vi "读取反控数据解析(子VI).vi"(6 "数据":string, 7 "命令编码CN":string) -> (2 "设置超时时间/min":i32=1, 3 "反控命令错误？":bool)   [LabVIEW 2016, in "数据传输系统-06.lvlib"]
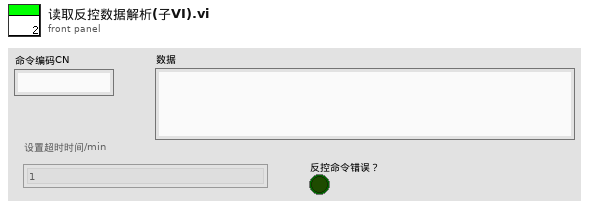
[diagram p1: front panel]
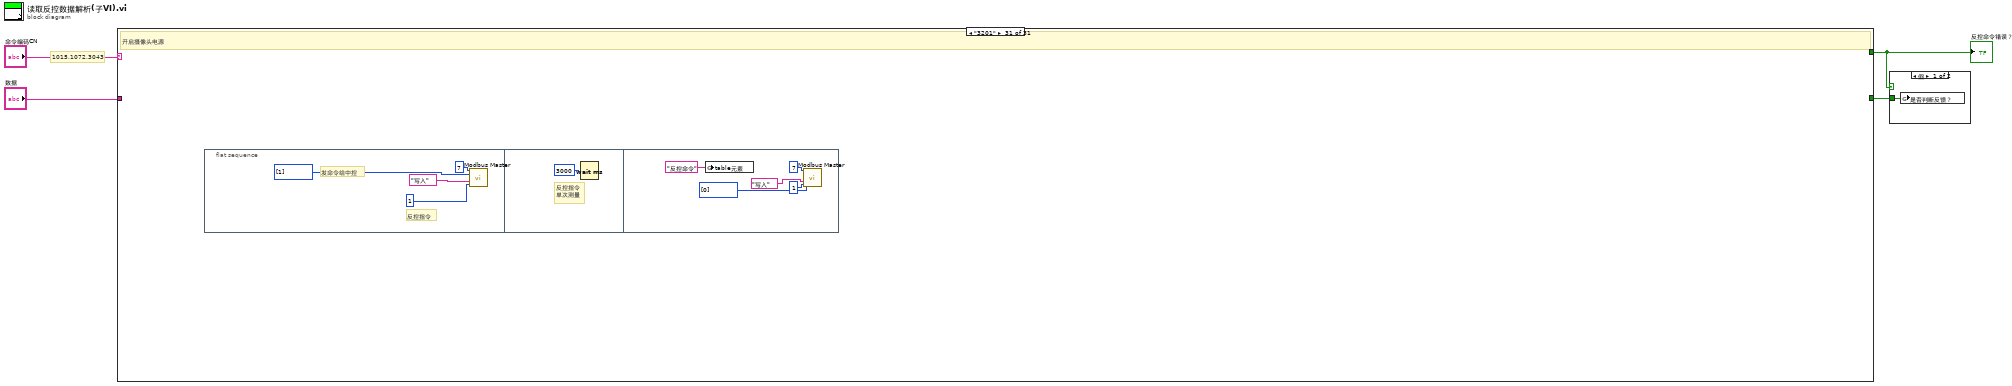
[diagram p0: block diagram]
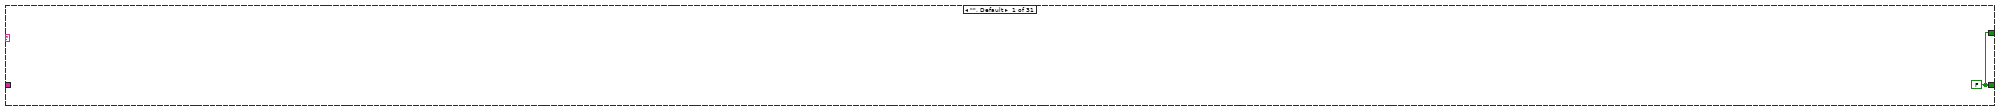
[diagram p2: hidden frame]
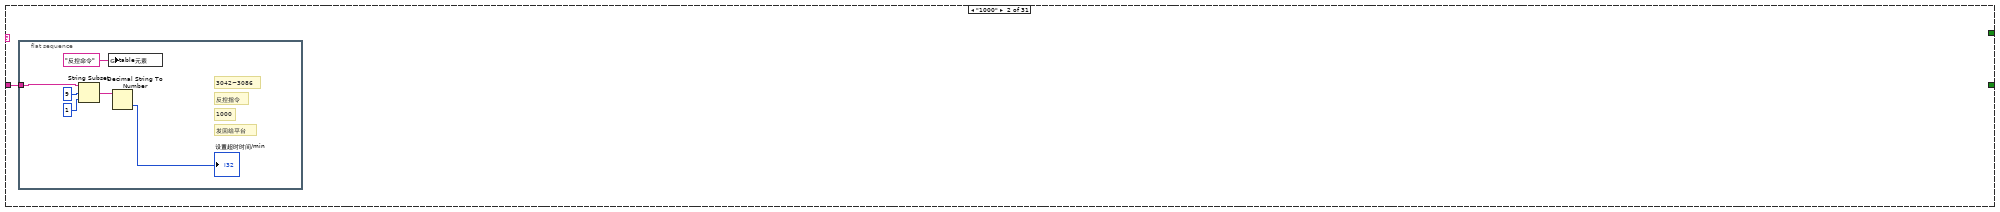
[diagram p3: hidden frame]
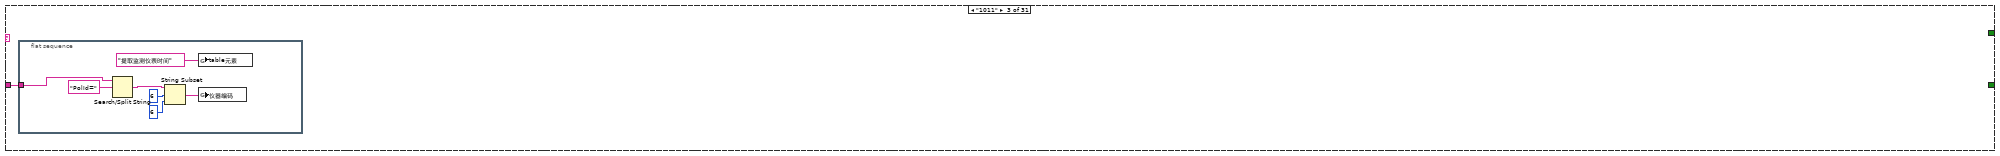
[diagram p4: hidden frame]
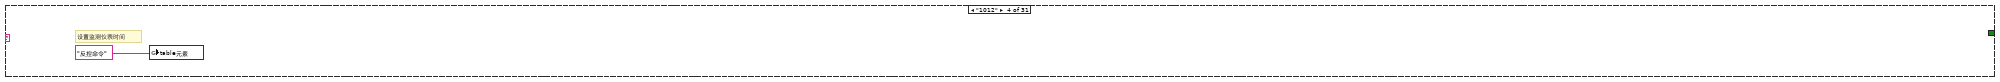
[diagram p5: hidden frame]
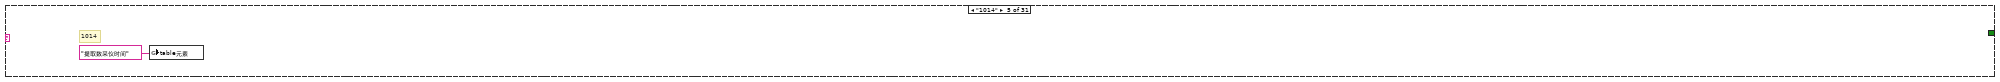
[diagram p6: hidden frame]
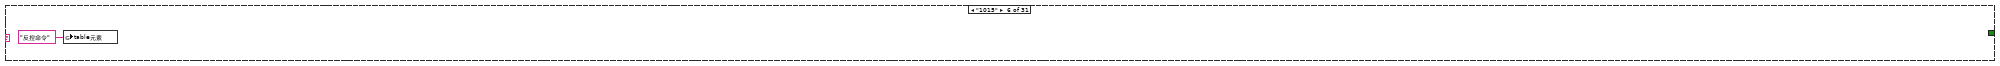
[diagram p7: hidden frame]
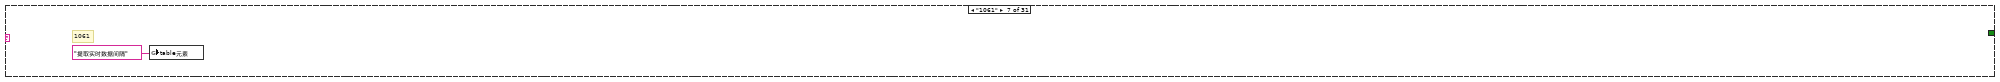
[diagram p8: hidden frame]
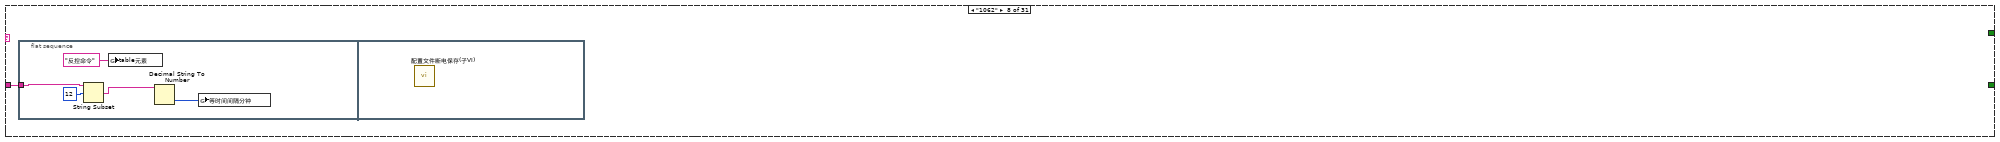
[diagram p9: hidden frame]
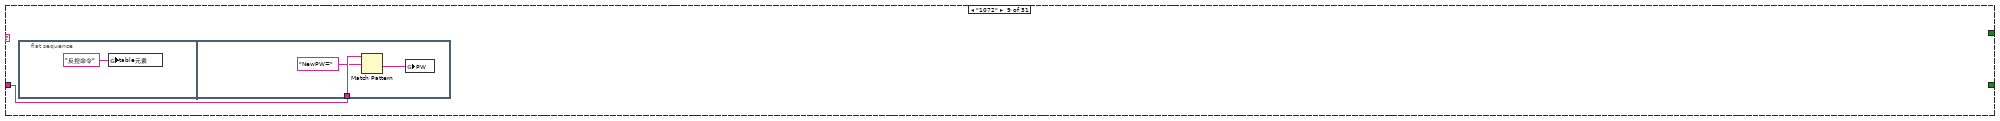
[diagram p10: hidden frame]
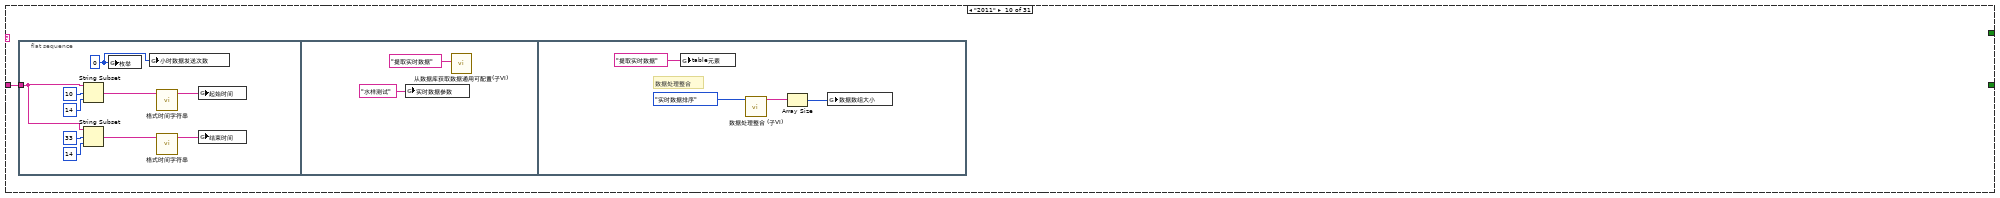
[diagram p11: hidden frame]
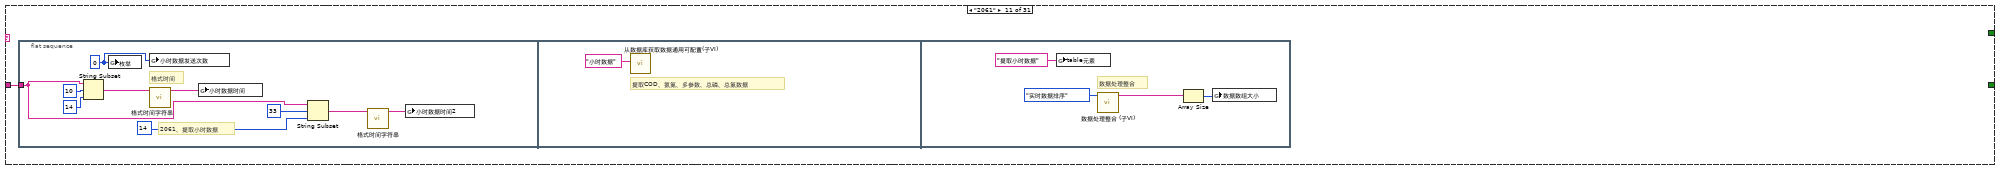
[diagram p12: hidden frame]
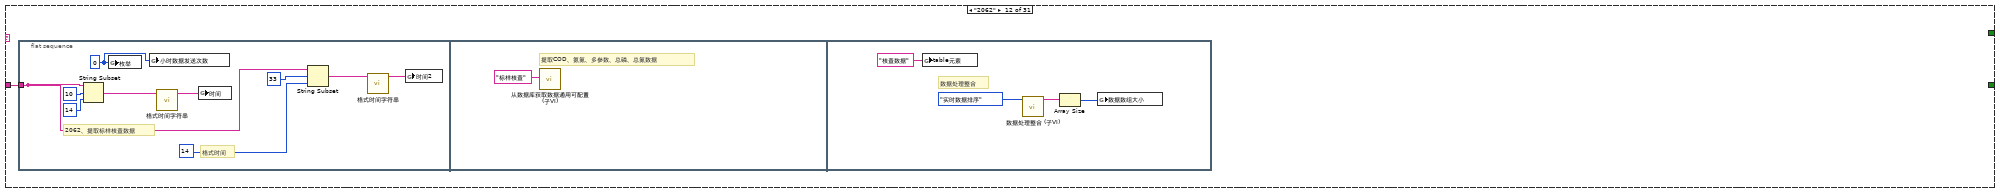
[diagram p13: hidden frame]
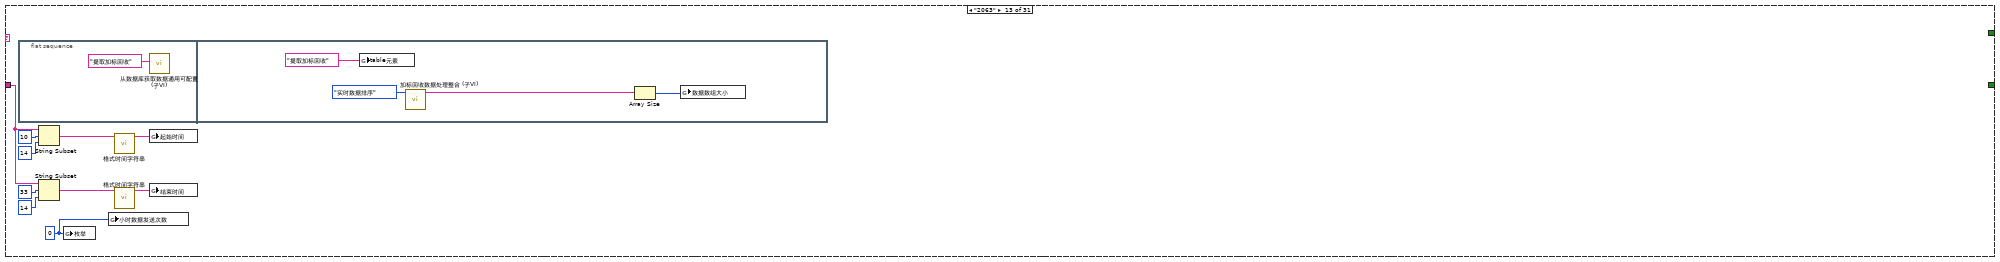
[diagram p14: hidden frame]
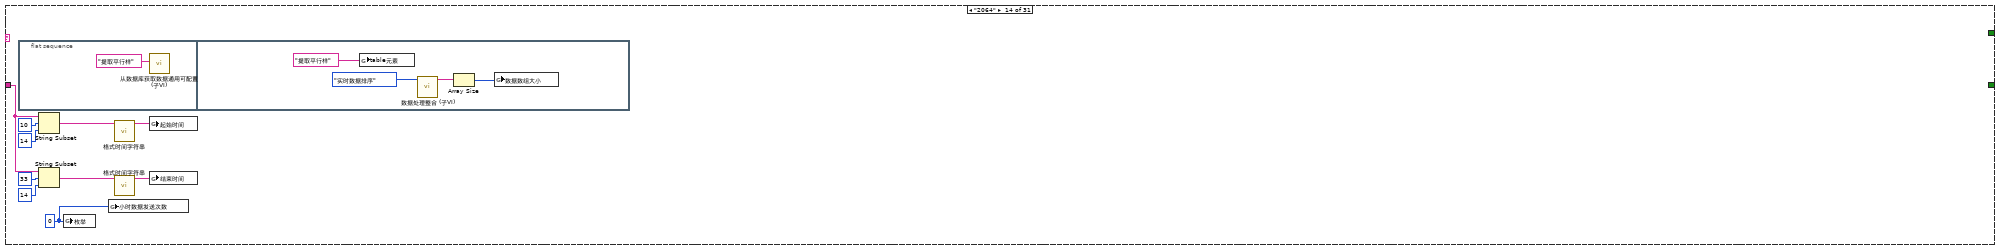
[diagram p15: hidden frame]
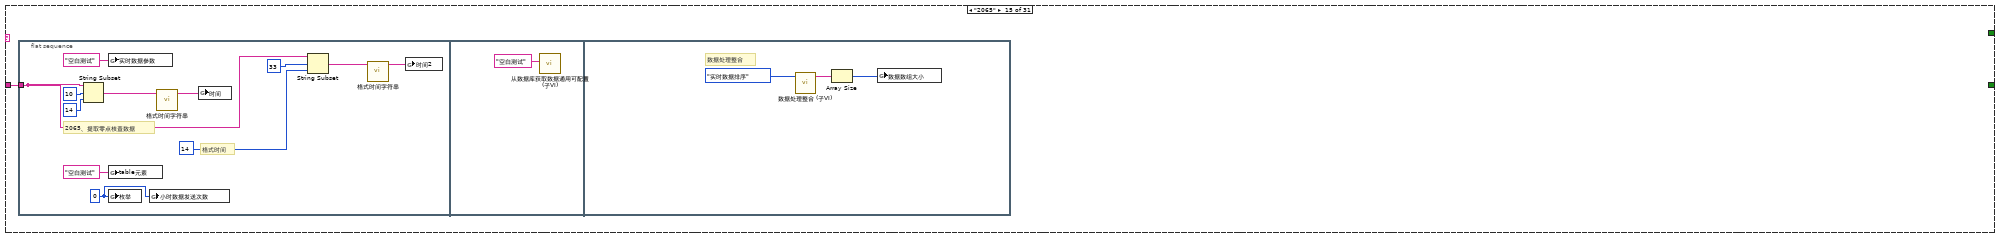
[diagram p16: hidden frame]
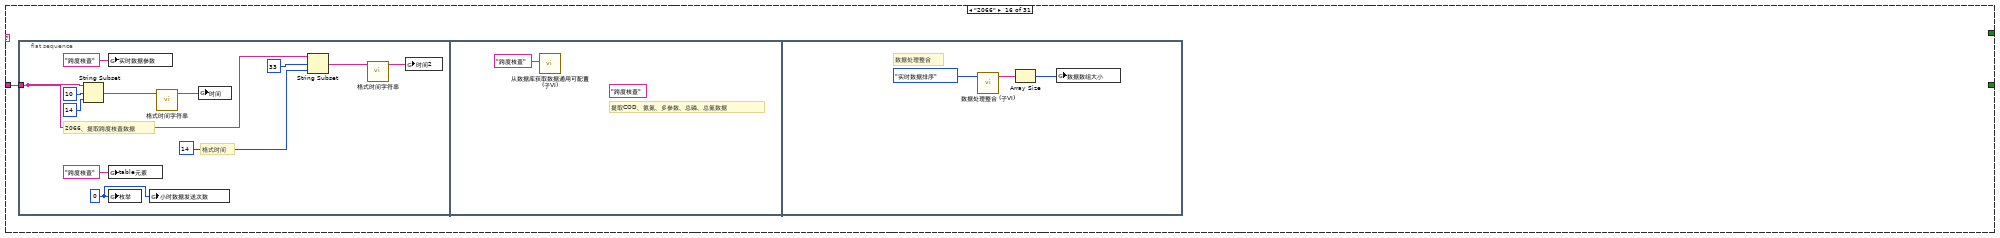
[diagram p17: hidden frame]
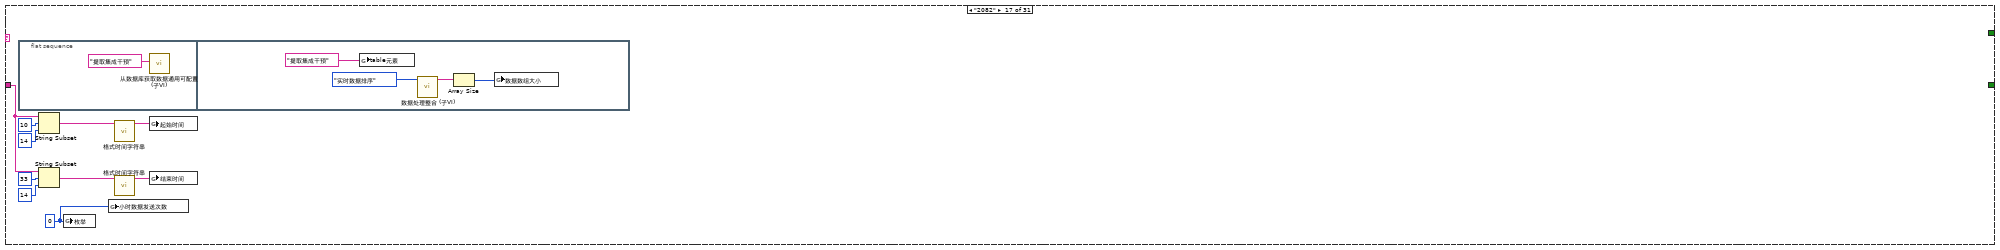
[diagram p18: hidden frame]
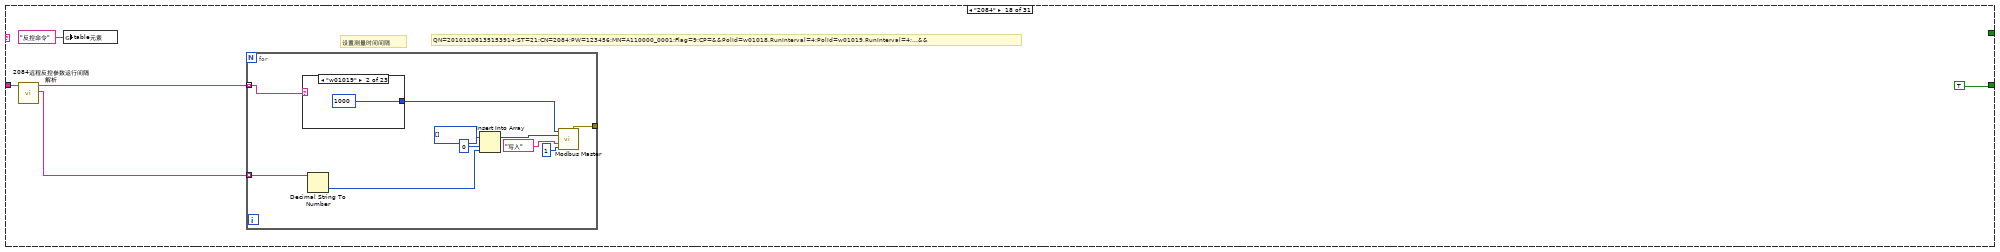
[diagram p19: hidden frame]
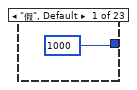
[diagram p20: hidden frame]
diagram:
  # "1015,1072,3043"
  n1 = case shown="\"3201\"" "命令编码CN" {
    selector: "命令编码CN" -> [_ _ _ _ _ _ _ _ _ _ _ _ _ _ _ _ _ _ _ _ _ _ _ _ _ _ _ _ w499 _ _]
    tunnel: "数据" -> [_ w6 w13 _ _ _ _ w25 w31 w36 w53 w69 w86 w100 w115 w132 w149 w165 _ w210 w367 _ _ w459 _ _ _ w498 w500 _ _]
    tunnel: [w5 _ _ _ _ _ _ _ _ _ _ _ _ _ _ _ _ _ _ _ _ _ _ _ _ _ _ _ _ _ _] -> w2
    tunnel: [w5 _ _ _ _ _ _ _ _ _ _ _ _ _ _ _ _ TRUE _ _ TRUE _ _ TRUE ("是否判断反馈？") _ _ _ _ TRUE _ _] -> w1
    frame "", Default {
      w5 = FALSE
    }
    frame "1000" {
      n2 = flat-sequence {
        tunnel: w6 -> [w8]
        frame #0 {
          # "发回给平台"
          # "3042~3086"
          # "反控指令"
          # "1000"
          n3 = String Subset(string=w8, offset (0)=9 ("偏移量(0)"), length (rest)=1 ("长度（剩余）")) -> (substring=w10:string)
          n4 = global write "全局1.vi" "table元素"("反控命令" ("新元素/子数组")) -> ()
          n5 = Decimal String To Number(string=w10) -> (number=→"设置超时时间/min":i32)  [unwired: 2 in, 1 out]
        }
      }
    }
    frame "1011" {
      n6 = flat-sequence {
        tunnel: w13 -> [w14]
        frame #0 {
          n7 = Search/Split String(string=w14, search string/char (-)="PolId=" ("搜索字符串/字符(-)")) -> (match + rest of string=w19:string)  [unwired: 1 in, 2 out]
          n8 = String Subset(string=w19, offset (0)=6 ("偏移量(0)"), length (rest)=6 ("长度（剩余）")) -> (substring=w16:string)
          n9 = global write "全局1.vi" "table元素"("提取监测仪表时间") -> ()
          n10 = global write "全局 提取仪器参数.vi" "仪器编码"(w16) -> ()
        }
      }
    }
    frame "1012" {
      # "设置监测仪表时间"
      n11 = global write "全局1.vi" "table元素"("反控命令" ("新元素/子数组")) -> ()
    }
    frame "1014" {
      # "1014"
      n12 = global write "全局1.vi" "table元素"("提取数采仪时间") -> ()
    }
    frame "1015" {
      n13 = global write "全局1.vi" "table元素"("反控命令" ("新元素/子数组")) -> ()
    }
    frame "1061" {
      # "1061"
      n14 = global write "全局1.vi" "table元素"("提取实时数据间隔") -> ()
    }
    frame "1062" {
      n15 = flat-sequence {
        tunnel: w25 -> [w28]
        frame #0 {
          n16 = String Subset(string=w28, offset (0)=12 ("偏移量(0)")) -> (substring=w29:string)  [unwired: 1 in]
          n17 = global write "全局1.vi" "table元素"("反控命令" ("新元素/子数组")) -> ()
          n18 = Decimal String To Number(string=w29) -> (number=w26:i32)  [unwired: 2 in, 1 out]
          n19 = global write "断电保存全局.vi" "等时间间隔分钟"(w26) -> ()
        }
        frame #1 {
          n20 = call "配置文件断电保存(子VI).vi"() -> ()  [unwired: 12 in]
        }
      }
    }
    frame "1072" {
      n21 = flat-sequence {
        tunnel: w31 -> [w35]
        frame #0 {
          n22 = global write "全局1.vi" "table元素"("反控命令" ("新元素/子数组")) -> ()
        }
        frame #1 {
          n23 = Match Pattern(string=w35, regular expression="NewPW=" ("正则表达式")) -> (after substring=w33:string)  [unwired: 1 in, 3 out]
          n24 = global write "断电保存全局.vi" "PW"(w33) -> ()
        }
      }
    }
    frame "2011" {
      n25 = flat-sequence {
        tunnel: w36 -> [w37]
        frame #0 {
          w42 = 0 ("数值")
          n26 = String Subset(string=w37, offset (0)=10 ("偏移量(0)"), length (rest)=14 ("长度（剩余）")) -> (substring=w45:string)
          n27 = String Subset(string=w37, offset (0)=33 ("偏移量(0)"), length (rest)=14 ("长度（剩余）")) -> (substring=w43:string)
          n28 = global write "全局1.vi" "枚举"(w42) -> ()
          n29 = global write "全局 小时数据发送次数.vi" "小时数据发送次数"(w42) -> ()
          n30 = call "格式时间字符串.vi"("字符串"=w45) -> ("连接的字符串"=w46:string)  [unwired: 10 in]
          n31 = call "格式时间字符串.vi"("字符串"=w43) -> ("连接的字符串"=w44:string)  [unwired: 10 in]
          n32 = global write "起始时间.vi" "起始时间"(w46) -> ()
          n33 = global write "起始时间.vi" "结束时间"(w44) -> ()
        }
        frame #1 {
          n34 = global write "全局 实时数据参数.vi" "实时数据参数"("水样测试") -> ()
          n35 = call "从数据库获取数据通用可配置(子VI).vi"("table输入"="提取实时数据" ("新元素/子数组")) -> ()  [unwired: 9 in, 2 out]
        }
        frame #2 {
          # "数据处理整合"
          n36 = global write "全局1.vi" "table元素"("提取实时数据" ("新元素/子数组")) -> ()
          n37 = call "数据处理整合 (子VI).vi"("枚举"=enum16{"实时数据排序", "小时数据排序"}."实时数据排序") -> ("已排序的数组"=w51:string[])  [unwired: 10 in]
          n38 = Array Size(array=w51) -> (size(s)=w52:i32)
          n39 = global write "全局 数据数组大小.vi" "数据数组大小"(w52) -> ()
        }
      }
    }
    frame "2061" {
      n40 = flat-sequence {
        tunnel: w53 -> [w54]
        frame #0 {
          w55 = 0 ("数值")
          # "格式时间"
          # "2061、提取小时数据"
          n41 = String Subset(string=w54, offset (0)=10 ("偏移量(0)"), length (rest)=14 ("长度（剩余）")) -> (substring=w58:string)
          n42 = global write "全局1.vi" "枚举"(w55) -> ()
          n43 = global write "全局 小时数据发送次数.vi" "小时数据发送次数"(w55) -> ()
          n44 = call "格式时间字符串.vi"("字符串"=w58) -> ("连接的字符串"=w59:string)  [unwired: 10 in]
          n45 = global write "全局 水样时间.vi" "小时数据时间"(w59) -> ()
          n46 = String Subset(string=w54, offset (0)=33 ("偏移量(0)"), length (rest)=14 ("长度（剩余）")) -> (substring=w57:string)
          n47 = call "格式时间字符串.vi"("字符串"=w57) -> ("连接的字符串"=w56:string)  [unwired: 10 in]
          n48 = global write "全局 时间2.vi" "小时数据时间2"(w56) -> ()
        }
        frame #1 {
          # "提取COD、氨氮、多参数、总磷、总氮数据"
          n49 = call "从数据库获取数据通用可配置(子VI).vi"("table输入"="小时数据" ("名称（未命名）")) -> ()  [unwired: 9 in, 2 out]
        }
        frame #2 {
          # "数据处理整合"
          n50 = global write "全局1.vi" "table元素"("提取小时数据" ("新元素/子数组")) -> ()
          n51 = call "数据处理整合 (子VI).vi"("枚举"=enum16{"实时数据排序", "小时数据排序"}."实时数据排序") -> ("已排序的数组"=w68:string[])  [unwired: 10 in]
          n52 = Array Size(array=w68) -> (size(s)=w67:i32)
          n53 = global write "全局 数据数组大小.vi" "数据数组大小"(w67) -> ()
        }
      }
    }
    frame "2062" {
      n54 = flat-sequence {
        tunnel: w69 -> [w70]
        frame #0 {
          w71 = 0 ("数值")
          # "格式时间"
          # "2062、提取标样核查数据"
          n55 = String Subset(string=w70, offset (0)=10 ("偏移量(0)"), length (rest)=14 ("长度（剩余）")) -> (substring=w74:string)
          n56 = global write "全局1.vi" "枚举"(w71) -> ()
          n57 = global write "全局 小时数据发送次数.vi" "小时数据发送次数"(w71) -> ()
          n58 = call "格式时间字符串.vi"("字符串"=w74) -> ("连接的字符串"=w75:string)  [unwired: 10 in]
          n59 = global write "全局 水样时间.vi" "时间"(w75) -> ()
          n60 = String Subset(string=w70, offset (0)=33 ("偏移量(0)"), length (rest)=14 ("长度（剩余）")) -> (substring=w73:string)
          n61 = call "格式时间字符串.vi"("字符串"=w73) -> ("连接的字符串"=w72:string)  [unwired: 10 in]
          n62 = global write "全局 时间2.vi" "时间2"(w72) -> ()
        }
        frame #1 {
          # "提取COD、氨氮、多参数、总磷、总氮数据"
          n63 = call "从数据库获取数据通用可配置(子VI).vi"("table输入"="标样核查" ("新元素/子数组")) -> ()  [unwired: 9 in, 2 out]
        }
        frame #2 {
          # "数据处理整合"
          n64 = global write "全局1.vi" "table元素"("核查数据" ("新元素/子数组")) -> ()
          n65 = call "数据处理整合 (子VI).vi"("枚举"=enum16{"实时数据排序", "小时数据排序"}."实时数据排序") -> ("已排序的数组"=w83:string[])  [unwired: 10 in]
          n66 = Array Size(array=w83) -> (size(s)=w84:i32)
          n67 = global write "全局 数据数组大小.vi" "数据数组大小"(w84) -> ()
        }
      }
    }
    frame "2063" {
      w85 = 0 ("数值")
      n68 = flat-sequence {
        frame #0 {
          n69 = call "从数据库获取数据通用可配置(子VI).vi"("table输入"="提取加标回收" ("新元素/子数组")) -> ()  [unwired: 9 in, 2 out]
        }
        frame #1 {
          n70 = global write "全局1.vi" "table元素"("提取加标回收" ("新元素/子数组")) -> ()
          n71 = call "加标回收数据处理整合 (子VI).vi"("枚举"=enum16{"实时数据排序", "小时数据排序"}."实时数据排序") -> ("已排序的数组"=w97:string[])  [unwired: 10 in]
          n72 = Array Size(array=w97) -> (size(s)=w99:i32)
          n73 = global write "全局 数据数组大小.vi" "数据数组大小"(w99) -> ()
        }
      }
      n74 = String Subset(string=w86, offset (0)=10 ("偏移量(0)"), length (rest)=14 ("长度（剩余）")) -> (substring=w88:string)
      n75 = String Subset(string=w86, offset (0)=33 ("偏移量(0)"), length (rest)=14 ("长度（剩余）")) -> (substring=w90:string)
      n76 = global write "全局1.vi" "枚举"(w85) -> ()
      n77 = global write "全局 小时数据发送次数.vi" "小时数据发送次数"(w85) -> ()
      n78 = call "格式时间字符串.vi"("字符串"=w88) -> ("连接的字符串"=w87:string)  [unwired: 10 in]
      n79 = call "格式时间字符串.vi"("字符串"=w90) -> ("连接的字符串"=w89:string)  [unwired: 10 in]
      n80 = global write "起始时间.vi" "起始时间"(w87) -> ()
      n81 = global write "起始时间.vi" "结束时间"(w89) -> ()
    }
    frame "2064" {
      w105 = 0 ("数值")
      n82 = flat-sequence {
        frame #0 {
          n83 = call "从数据库获取数据通用可配置(子VI).vi"("table输入"="提取平行样" ("新元素/子数组")) -> ()  [unwired: 9 in, 2 out]
        }
        frame #1 {
          n84 = global write "全局1.vi" "table元素"("提取平行样" ("新元素/子数组")) -> ()
          n85 = call "数据处理整合 (子VI).vi"("枚举"=enum16{"实时数据排序", "小时数据排序"}."实时数据排序") -> ("已排序的数组"=w114:string[])  [unwired: 10 in]
          n86 = Array Size(array=w114) -> (size(s)=w113:i32)
          n87 = global write "全局 数据数组大小.vi" "数据数组大小"(w113) -> ()
        }
      }
      n88 = String Subset(string=w100, offset (0)=10 ("偏移量(0)"), length (rest)=14 ("长度（剩余）")) -> (substring=w108:string)
      n89 = String Subset(string=w100, offset (0)=33 ("偏移量(0)"), length (rest)=14 ("长度（剩余）")) -> (substring=w106:string)
      n90 = global write "全局1.vi" "枚举"(w105) -> ()
      n91 = global write "全局 小时数据发送次数.vi" "小时数据发送次数"(w105) -> ()
      n92 = call "格式时间字符串.vi"("字符串"=w108) -> ("连接的字符串"=w109:string)  [unwired: 10 in]
      n93 = call "格式时间字符串.vi"("字符串"=w106) -> ("连接的字符串"=w107:string)  [unwired: 10 in]
      n94 = global write "起始时间.vi" "起始时间"(w109) -> ()
      n95 = global write "起始时间.vi" "结束时间"(w107) -> ()
    }
    frame "2065" {
      n96 = flat-sequence {
        tunnel: w115 -> [w117]
        frame #0 {
          w118 = 0 ("数值")
          # "格式时间"
          # "2065、提取零点核查数据"
          n97 = String Subset(string=w117, offset (0)=10 ("偏移量(0)"), length (rest)=14 ("长度（剩余）")) -> (substring=w122:string)
          n98 = global write "全局 实时数据参数.vi" "实时数据参数"("空白测试" ("新元素/子数组")) -> ()
          n99 = global write "全局1.vi" "table元素"("空白测试" ("新元素/子数组")) -> ()
          n100 = global write "全局1.vi" "枚举"(w118) -> ()
          n101 = global write "全局 小时数据发送次数.vi" "小时数据发送次数"(w118) -> ()
          n102 = call "格式时间字符串.vi"("字符串"=w122) -> ("连接的字符串"=w123:string)  [unwired: 10 in]
          n103 = global write "全局 水样时间.vi" "时间"(w123) -> ()
          n104 = String Subset(string=w117, offset (0)=33 ("偏移量(0)"), length (rest)=14 ("长度（剩余）")) -> (substring=w121:string)
          n105 = call "格式时间字符串.vi"("字符串"=w121) -> ("连接的字符串"=w120:string)  [unwired: 10 in]
          n106 = global write "全局 时间2.vi" "时间2"(w120) -> ()
        }
        frame #1 {
          n107 = call "从数据库获取数据通用可配置(子VI).vi"("table输入"="空白测试" ("新元素/子数组")) -> ()  [unwired: 9 in, 2 out]
        }
        frame #2 {
          # "数据处理整合"
          n108 = call "数据处理整合 (子VI).vi"("枚举"=enum16{"实时数据排序", "小时数据排序"}."实时数据排序") -> ("已排序的数组"=w130:string[])  [unwired: 10 in]
          n109 = Array Size(array=w130) -> (size(s)=w131:i32)
          n110 = global write "全局 数据数组大小.vi" "数据数组大小"(w131) -> ()
        }
      }
    }
    frame "2066" {
      n111 = flat-sequence {
        tunnel: w132 -> [w134]
        frame #0 {
          w135 = 0 ("数值")
          # "格式时间"
          # "2066、提取跨度核查数据"
          n112 = String Subset(string=w134, offset (0)=10 ("偏移量(0)"), length (rest)=14 ("长度（剩余）")) -> (substring=w139:string)
          n113 = global write "全局 实时数据参数.vi" "实时数据参数"("跨度核查" ("新元素/子数组")) -> ()
          n114 = global write "全局1.vi" "table元素"("跨度核查" ("新元素/子数组")) -> ()
          n115 = global write "全局1.vi" "枚举"(w135) -> ()
          n116 = global write "全局 小时数据发送次数.vi" "小时数据发送次数"(w135) -> ()
          n117 = call "格式时间字符串.vi"("字符串"=w139) -> ("连接的字符串"=w140:string)  [unwired: 10 in]
          n118 = global write "全局 水样时间.vi" "时间"(w140) -> ()
          n119 = String Subset(string=w134, offset (0)=33 ("偏移量(0)"), length (rest)=14 ("长度（剩余）")) -> (substring=w138:string)
          n120 = call "格式时间字符串.vi"("字符串"=w138) -> ("连接的字符串"=w137:string)  [unwired: 10 in]
          n121 = global write "全局 时间2.vi" "时间2"(w137) -> ()
        }
        frame #1 {
          (unwired) "跨度核查" ("名称（未命名）")
          # "提取COD、氨氮、多参数、总磷、总氮数据"
          n122 = call "从数据库获取数据通用可配置(子VI).vi"("table输入"="跨度核查" ("新元素/子数组")) -> ()  [unwired: 9 in, 2 out]
        }
        frame #2 {
          # "数据处理整合"
          n123 = call "数据处理整合 (子VI).vi"("枚举"=enum16{"实时数据排序", "小时数据排序"}."实时数据排序") -> ("已排序的数组"=w148:string[])  [unwired: 10 in]
          n124 = Array Size(array=w148) -> (size(s)=w147:i32)
          n125 = global write "全局 数据数组大小.vi" "数据数组大小"(w147) -> ()
        }
      }
    }
    frame "2082" {
      w154 = 0 ("数值")
      n126 = flat-sequence {
        frame #0 {
          n127 = call "从数据库获取数据通用可配置(子VI).vi"("table输入"="提取集成干预" ("新元素/子数组")) -> ()  [unwired: 9 in, 2 out]
        }
        frame #1 {
          n128 = global write "全局1.vi" "table元素"("提取集成干预" ("新元素/子数组")) -> ()
          n129 = call "数据处理整合 (子VI).vi"("枚举"=enum16{"实时数据排序", "小时数据排序"}."实时数据排序") -> ("已排序的数组"=w163:string[])  [unwired: 10 in]
          n130 = Array Size(array=w163) -> (size(s)=w162:i32)
          n131 = global write "全局 数据数组大小.vi" "数据数组大小"(w162) -> ()
        }
      }
      n132 = String Subset(string=w149, offset (0)=10 ("偏移量(0)"), length (rest)=14 ("长度（剩余）")) -> (substring=w157:string)
      n133 = String Subset(string=w149, offset (0)=33 ("偏移量(0)"), length (rest)=14 ("长度（剩余）")) -> (substring=w155:string)
      n134 = global write "全局1.vi" "枚举"(w154) -> ()
      n135 = global write "全局 小时数据发送次数.vi" "小时数据发送次数"(w154) -> ()
      n136 = call "格式时间字符串.vi"("字符串"=w157) -> ("连接的字符串"=w158:string)  [unwired: 10 in]
      n137 = call "格式时间字符串.vi"("字符串"=w155) -> ("连接的字符串"=w156:string)  [unwired: 10 in]
      n138 = global write "起始时间.vi" "起始时间"(w158) -> ()
      n139 = global write "起始时间.vi" "结束时间"(w156) -> ()
    }
    frame "2084" {
      # "设置测量时间间隔"
      # "QN=20101108135153914;ST=21;CN=2084;PW=123456;MN=A110000_0001;Flag=9;CP=&&PolId=w01018,RunInterval=4;PolId=w01019,RunInterval=4;...&&"
      n140 = call "2084远程反控参数运行间隔解析.vi"("字符串"=w165) -> ("Value"=w168:string[], "因子编码"=w167:string[])  [unwired: 9 in]
      n141 = global write "全局1.vi" "table元素"("反控命令" ("新元素/子数组")) -> ()
      n142 = for {
        tunnel: w167 -> [w174] mode=indexing
        tunnel: w168 -> [w178] mode=indexing
        tunnel: [w169] -> _
        n143 = case shown="\"w01019\"" w174 {
          tunnel: [1000 1000 1001 1002 1003 1004 1005 1006 1007 1008 1009 1010 1011 1012 1013 1014 1015 1016 1017 1018 1019 1020 1021] -> w170
          frame "假", Default {
          }
          frame "w01019" {
          }
          frame "w01018" {
          }
          frame "w01009" {
          }
          frame "w01001" {
          }
          frame "w21003" {
          }
          frame "w01014" {
          }
          frame "w01010" {
          }
          frame "w01003" {
          }
          frame "w21001" {
          }
          frame "w21011" {
          }
          frame "w01016" {
          }
          frame "w19011" {
          }
          frame "w21006" {
          }
          frame "w21019" {
          }
          frame "w01100" {
          }
          frame "w20120" {
          }
          frame "w20115" {
          }
          frame "w20122" {
          }
          frame "w20123" {
          }
          frame "w20121" {
          }
          frame "w20124" {
          }
          frame "w20111" {
          }
        }
        n144 = Decimal String To Number(string=w178) -> (number=w175:i32)  [unwired: 2 in, 1 out]
        n145 = Insert Into Array(array=u16[] [] ("holding register values"), index=0 ("索引"), new element=w175) -> (w173:u16[])
        n146 = call "Modbus Master.vi"("starting address"=w170, "holding register values"=w173, "读取写入选择"="写入", "Unit ID"=u8 1) -> ("error out"=w169:errorcluster)  [unwired: 6 in, 5 out]
      }
    }
    frame "3015" {
      n147 = flat-sequence {
        frame #0 {
          # "发命令给中控"
          # "发回给平台"
          # "3015、手动远程留样"
          n148 = global write "全局1.vi" "table元素"("超标留样返回" ("新元素/子数组")) -> ()
          n149 = Insert Into Array(array=u16[] [] ("holding register values"), index=0 ("索引"), new element=u16 1 ("新元素/子数组")) -> (w205:u16[])
          n150 = call "Modbus Master.vi"("starting address"=u16 10, "holding register values"=w205, "读取写入选择"="写入", "Unit ID"=u8 1) -> ()  [unwired: 6 in, 6 out]
        }
      }
    }
    frame "3020" {
      n151 = flat-sequence {
        tunnel: [w222] -> w216
        tunnel: [w223] -> w215
        tunnel: [w219] -> w214
        tunnel: [w221] -> w213
        tunnel: w210 -> [w220]
        tunnel: [w220] -> w212
        tunnel: w216 -> [w251]
        tunnel: w215 -> [w252]
        tunnel: w214 -> [w253]
        tunnel: w213 -> [w255]
        tunnel: [w254] -> w211
        tunnel: w212 -> [w254]
        tunnel: w211 -> [w339]
        frame #0 {
          w217 = "操作日志报警信息" ("名称（未命名）")
          w226 = 0 ("数值")
          # "3020、提取日志、报警，仪器参数"
          n152 = call "日志报警参数选择 (子VI).vi"("String输入"=w220) -> ("输出boll数组"=w218:bool[], "输出char数组"=w219:string[])  [unwired: 7 in, 2 out]
          n153 = global write "全局1.vi" "枚举"(w226) -> ()
          n154 = global write "全局 小时数据发送次数.vi" "小时数据发送次数"(w226) -> ()
          n155 = Search/Split String(string=w220, search string/char (-)="BeginTime=" ("搜索字符串")) -> (match + rest of string=w225:string)  [unwired: 1 in, 2 out]
          n156 = case shown="\"\"" w225 {
            tunnel: ["1904/01/01 00:00:00" w248] -> w228
            tunnel: w225 -> [_ w242]
            tunnel: [w236 w243] -> w224
            frame "" {
              n157 = Get Date/Time In Seconds() -> (seconds since 1Jan1904=w238:timestamp)
              n158 = Format Date/Time String(time format string (%c)="%Y/%m/%d %H:%M:%S" ("时间格式字符串(%c)"), seconds (now)=w238) -> (date/time string=w239:string)  [unwired: 1 in]
              n159 = Search and Replace String(input string=w239, search string="." ("搜索字符串")) -> (result string=w236:string)  [unwired: 6 in, 3 out]
            }
            frame "真", Default {
              # "格式时间"
              n160 = String Subset(string=w242, offset (0)=10 ("偏移量(0)"), length (rest)=14 ("长度（剩余）")) -> (substring=w247:string)
              n161 = String Subset(string=w242, offset (0)=33 ("偏移量(0)"), length (rest)=14 ("长度（剩余）")) -> (substring=w246:string)
              n162 = call "格式时间字符串.vi"("字符串"=w247) -> ("连接的字符串"=w248:string)  [unwired: 10 in]
              n163 = call "格式时间字符串.vi"("字符串"=w246) -> ("连接的字符串"=w243:string)  [unwired: 10 in]
            }
          }
          n164 = Or Array Elements(Boolean array=w218) -> (logical OR=w221:bool)
          n165 = Obtain Queue(name (unnamed)=w217, element data type=w217) -> (queue out=w222:refnum<queue>, error out=w223:errorcluster)  [unwired: 3 in, 1 out]
          n166 = case shown="真" w221 {
            tunnel: w222 -> [_ w230]
            tunnel: w218 -> [_ w229]
            frame False {
            }
            frame True {
              n167 = for {
                tunnel: w229 -> [w232] mode=indexing
                tunnel: w230 -> [w231]
                i -> [w233]
                n168 = case shown="真" w232 {
                  tunnel: w233 -> [_ w235]
                  tunnel: w231 -> [_ w234]
                  frame False {
                  }
                  frame True {
                    n169 = call "提取日志报警参数入列队 (子VI).vi"("索引"=w235, "队列输入"=w234) -> ()  [unwired: 10 in]
                  }
                }
              }
            }
          }
          n170 = global write "全局 水样时间.vi" "时间"(w228) -> ()
          n171 = global write "全局 时间2.vi" "时间2"(w224) -> ()
        }
        frame #1 {
          # "按需求提取COD、氨氮、总磷、总氮日志"
          # "按需求提取COD、氨氮、总磷、总氮日志"
          n172 = case shown="真" w255 {
            tunnel: w252 -> [_ w258]
            tunnel: w251 -> [_ w257]
            tunnel: w253 -> [_ w256]
            frame False {
            }
            frame True {
              n173 = while {
                shift-right: [w259] -> _
                shift-left: w257 -> [w267]
                tunnel: w258 -> [w266]
                tunnel: w256 -> [w260]
                stop <- w263 stop-if-true
                n174 = Dequeue Element(queue=w267, error in (no error)=w266) -> (queue out=w265:refnum<queue>, element=w261:string)  [unwired: 1 in, 2 out]
                n175 = Wait (ms)(milliseconds to wait=u32 300 ("等待时间（毫秒）")) -> ()  [unwired: 1 out]
                n176 = case shown="\"CODMn\", 默认" w261 {
                  tunnel: w265 -> [_ _ _ _ _ _ _ _ _ _ _ _ _ _]
                  tunnel: w260 -> [w269 w274 w279 w284 w289 w295 w298 w303 w308 w313 w318 w323 w328 w333]
                  frame "CODMn", Default {
                    n177 = Index Array(array=w269, index=0 ("索引")) -> (element=w268:string)
                    n178 = call "数据表比对.vi"("仪器日志参数"="CODMn" ("元素"), "table输入"=w268) -> ("待发送数据"=w271:string[][])  [unwired: 6 in, 3 out]
                    n179 = global write "全局 所有参数.vi" "CODMn"(w271) -> ()
                  }
                  frame "CODCr" {
                    n180 = Index Array(array=w274, index=1 ("索引")) -> (element=w273:string)
                    n181 = call "数据表比对.vi"("仪器日志参数"="CODCr" ("元素"), "table输入"=w273) -> ("待发送数据"=w276:string[][])  [unwired: 6 in, 3 out]
                    n182 = global write "全局 所有参数.vi" "CODCr"(w276) -> ()
                  }
                  frame "氨氮" {
                    n183 = Index Array(array=w279, index=2 ("索引")) -> (element=w278:string)
                    n184 = call "数据表比对.vi"("仪器日志参数"="氨氮" ("元素"), "table输入"=w278) -> ("待发送数据"=w281:string[][])  [unwired: 6 in, 3 out]
                    n185 = global write "全局 所有参数.vi" "氨氮"(w281) -> ()
                  }
                  frame "总磷" {
                    n186 = Index Array(array=w284, index=3 ("索引")) -> (element=w283:string)
                    n187 = call "数据表比对.vi"("仪器日志参数"="总磷" ("元素"), "table输入"=w283) -> ("待发送数据"=w286:string[][])  [unwired: 6 in, 3 out]
                    n188 = global write "全局 所有参数.vi" "总磷"(w286) -> ()
                  }
                  frame "总氮" {
                    n189 = Index Array(array=w289, index=4 ("索引")) -> (element=w288:string)
                    n190 = call "数据表比对.vi"("仪器日志参数"="总氮" ("元素"), "table输入"=w288) -> ("待发送数据"=w291:string[][])  [unwired: 6 in, 3 out]
                    n191 = global write "全局 所有参数.vi" "总氮"(w291) -> ()
                  }
                  frame "数采仪" {
                    n192 = Index Array(array=w295, index=5 ("索引")) -> (element=w293:string)
                    n193 = call "数据表比对.vi"("仪器日志参数"="系统" ("元素"), "table输入"=w293) -> ("待发送数据"=w296:string[][])  [unwired: 6 in, 3 out]
                    n194 = global write "全局 所有参数.vi" "DO"(w296) -> ()
                  }
                  frame "PH" {
                    n195 = Index Array(array=w298, index=6 ("索引")) -> (element=w299:string)
                    n196 = call "数据表比对.vi"("仪器日志参数"="PH" ("元素"), "table输入"=w299) -> ("待发送数据"=w301:string[][])  [unwired: 6 in, 3 out]
                    n197 = global write "全局 所有参数.vi" "PH"(w301) -> ()
                  }
                  frame "电导率" {
                    n198 = Index Array(array=w303, index=7 ("索引")) -> (element=w304:string)
                    n199 = call "数据表比对.vi"("仪器日志参数"="电导率" ("元素"), "table输入"=w304) -> ("待发送数据"=w306:string[][])  [unwired: 6 in, 3 out]
                    n200 = global write "全局 所有参数.vi" "电导率"(w306) -> ()
                  }
                  frame "水温" {
                    n201 = Index Array(array=w308, index=8 ("索引")) -> (element=w309:string)
                    n202 = call "数据表比对.vi"("仪器日志参数"="水温" ("元素"), "table输入"=w309) -> ("待发送数据"=w311:string[][])  [unwired: 6 in, 3 out]
                    n203 = global write "全局 所有参数.vi" "水温"(w311) -> ()
                  }
                  frame "DO" {
                    n204 = Index Array(array=w313, index=9 ("索引")) -> (element=w314:string)
                    n205 = call "数据表比对.vi"("仪器日志参数"="溶解氧" ("元素"), "table输入"=w314) -> ("待发送数据"=w316:string[][])  [unwired: 6 in, 3 out]
                    n206 = global write "全局 所有参数.vi" "DO"(w316) -> ()
                  }
                  frame "浊度" {
                    n207 = Index Array(array=w318, index=10 ("索引")) -> (element=w319:string)
                    n208 = call "数据表比对.vi"("仪器日志参数"="浊度" ("元素"), "table输入"=w319) -> ("待发送数据"=w321:string[][])  [unwired: 6 in, 3 out]
                    n209 = global write "全局 所有参数.vi" "浊度"(w321) -> ()
                  }
                  frame "叶绿素" {
                    n210 = Index Array(array=w323, index=11 ("索引")) -> (element=w324:string)
                    n211 = call "数据表比对.vi"("仪器日志参数"="叶绿素" ("元素"), "table输入"=w324) -> ("待发送数据"=w326:string[][])  [unwired: 6 in, 3 out]
                    n212 = global write "全局 所有参数.vi" "叶绿素"(w326) -> ()
                  }
                  frame "藻密度" {
                    n213 = Index Array(array=w328, index=12 ("索引")) -> (element=w329:string)
                    n214 = call "数据表比对.vi"("仪器日志参数"="藻密度" ("元素"), "table输入"=w329) -> ("待发送数据"=w331:string[][])  [unwired: 6 in, 3 out]
                    n215 = global write "全局 所有参数.vi" "藻密度"(w331) -> ()
                  }
                  frame "ORP" {
                    n216 = Index Array(array=w333, index=13 ("索引")) -> (element=w334:string)
                    n217 = call "数据表比对.vi"("仪器日志参数"="ORP" ("元素"), "table输入"=w334) -> ("待发送数据"=w336:string[][])  [unwired: 6 in, 3 out]
                    n218 = global write "全局 所有参数.vi" "ORP"(w336) -> ()
                  }
                }
                n219 = Get Queue Status(queue=w265) -> (queue out=w259:refnum<queue>, # elements in queue=w264:i32)  [unwired: 2 in, 6 out]
                n220 = Equal To 0?(x=w264) -> (x = 0?=w263:bool)
              }
            }
          }
        }
        frame #2 {
          w348 = "InfoId=" ("搜索字符串/字符(-)")
          n221 = Spreadsheet String To Array(delimiter (Tab)=";" ("分隔符(Tab)"), format string="" ("格式字符串"), spreadsheet string=w339, array type (2D Dbl)=string[] []) -> (array=w340:string[])
          n222 = Index Array(array=w340) -> (element=w338:string)  [unwired: 1 in]
          n223 = Search/Split String(string=w338, search string/char (-)=w348) -> (match + rest of string=w347:string)  [unwired: 1 in, 2 out]
          n224 = Search and Replace String(replace all?=TRUE ("替换全部？(F)"), input string=w347, search string=w348, replace string="" ("替换字符串(\"\")")) -> (result string=w344:string)  [unwired: 4 in, 3 out]
          n225 = Spreadsheet String To Array(delimiter (Tab)="," ("分隔符(Tab)"), format string="" ("格式字符串"), spreadsheet string=w344, array type (2D Dbl)=string[] []) -> (array=w346:string[])
          n226 = Index Array(array=w346) -> (element=w345:string)  [unwired: 1 in]
          n227 = case shown="默认" w345 {
            tunnel: ["操作日志" ("名称（未命名）") "提取仪器参数" ("名称（未命名）") "报警信息" ("名称（未命名）") "" ("名称（未命名）")] -> w354
            tunnel: [w356 1 ("数据数组大小") 1 _] -> w355
            tunnel: w344 -> [_ w360 _ _]
            frame "i11001", "i21001" {
              # "数据处理整合"
              # "i11001日志"
              n228 = call "数据处理整合 (子VI).vi"("枚举"=enum16{"实时数据排序", "小时数据排序"}."实时数据排序") -> ("已排序的数组"=w357:string[])  [unwired: 10 in]
              n229 = Array Size(array=w357) -> (size(s)=w356:i32)
            }
            frame "i13001", "i13002", "i13003", "i13004", "i13005", "i13006", "i13007", "i13008", "i13009", "i13010", "i13011", "i13012", "i13013", "i13014", "i13015", "i13016", "i13017", "i13101", "i13102", "i13103", "i13104", "i13105", "i13106", "i13107", "i13108", "i13109", "i13110" {
              n230 = call "数据处理直接插入整合 (子VI).vi"() -> ()  [unwired: 12 in]
              n231 = global write "全局 提取仪器参数.vi" "参数编码"(w360) -> ()
            }
            frame "i12001" {
              # "i12001状态"
              n232 = call "数据处理直接插入整合 (子VI).vi"() -> ()  [unwired: 12 in]
            }
            frame Default {
            }
          }
          n233 = global write "全局1.vi" "table元素"(w354) -> ()
          n234 = global write "全局 数据数组大小.vi" "数据数组大小"(w355) -> ()
        }
      }
    }
    frame "3021" {
      n235 = call "设置仪器参数命令解析.vi"("String输入"=w367) -> ("设置参数信息数组"=w368:string[][])  [unwired: 9 in, 1 out]
      n236 = for {
        tunnel: w368 -> [w371] mode=indexing
        # "同时设置几个参数?"
        n237 = flat-sequence {
          tunnel: w371 -> [w381]
          tunnel: [w372] -> w369
          tunnel: [w433] -> w370
          tunnel: w369 -> [w433]
          tunnel: w370 -> [w437]
          frame #0 {
            # "设置仪表参数"
            # "3|4个字节"
            # "反控指令"
            # "发命令给中控"
            # "1.因子编码\n2.关键参数\n3.值"
            n238 = Index Array(array=w381) -> (element #1=w380:string, element #2=w377:string, element #3=w376:string)  [unwired: 3 in]
            n239 = case shown="\"w01001\"" w380 {
              tunnel: [u16 0 ("starting address") u16 1 ("starting address") u16 2 ("starting address") u16 3 ("starting address") u16 4 ("starting address") u16 5 ("starting address") u16 6 ("starting address") u16 7 ("starting address") u16 8 ("starting address") u16 9 ("starting address") u16 10 ("starting address") u16 11 ("starting address") u16 12 ("starting address") u16 13 ("starting address")] -> w375
              frame "", Default {
              }
              frame "w01019" {
              }
              frame "w01001" {
              }
              frame "w21003" {
              }
              frame "w21001" {
              }
              frame "w21011" {
              }
              frame "w01018" {
              }
              frame "w01014" {
              }
              frame "w01010" {
              }
              frame "w01009" {
              }
              frame "w01003" {
              }
              frame "w01016" {
              }
              frame "w19011" {
              }
              frame "w01100" {
              }
            }
            n240 = case shown="\"i13101\"" w377 {
              tunnel: [u16 256 ("starting address") u16 256 ("starting address") u16 260 ("starting address") u16 264 ("starting address") u16 268 ("starting address") u16 272 ("starting address") u16 276 ("starting address") u16 280 ("starting address") u16 284 ("starting address") u16 288 ("starting address") u16 292 ("starting address") u16 296 ("starting address") u16 300 ("starting address") u16 304 ("starting address") u16 308 ("starting address") u16 312 ("starting address") u16 316 ("starting address") u16 320 ("starting address") u16 356 ("starting address") u16 360 ("starting address") u16 364 ("starting address") u16 368 ("starting address") u16 372 ("starting address") u16 376 ("starting address") u16 380 ("starting address") u16 384 ("starting address") u16 388 ("starting address") u16 392 ("starting address")] -> w372
              frame "", Default {
              }
              frame "i13001" {
              }
              frame "i13002" {
              }
              frame "i13003" {
              }
              frame "i13004" {
              }
              frame "i13005" {
              }
              frame "i13006" {
              }
              frame "i13007" {
              }
              frame "i13008" {
              }
              frame "i13009" {
              }
              frame "i13010" {
              }
              frame "i13011" {
              }
              frame "i13012" {
              }
              frame "i13013" {
              }
              frame "i13014" {
              }
              frame "i13015" {
              }
              frame "i13016" {
              }
              frame "i13017" {
              }
              frame "i13101" {
              }
              frame "i13102" {
              }
              frame "i13103" {
              }
              frame "i13104" {
              }
              frame "i13105" {
              }
              frame "i13106" {
              }
              frame "i13107" {
              }
              frame "i13108" {
              }
              frame "i13109" {
              }
              frame "i13110" {
              }
            }
            n241 = case shown="\"i13006\", \"i13013\"" w377 {
              tunnel: w376 -> [w385 w390]
              tunnel: [w383 w386] -> w374
              frame "假", Default {
                n242 = Fract/Exp String To Number(string=w385) -> (number=w382:dbl)  [unwired: 3 in, 1 out]
                n243 = Build Array(w382) -> (w384:dbl[])
                n244 = call "FloatToHex.vi"("浮点数"=w384) -> ("DCBA整形输出"=w383:u16[])  [unwired: 10 in]
              }
              frame "i13006", "i13013" {
                n245 = call "格式时间字符串.vi"("字符串"=w390) -> ("连接的字符串"=w389:string)  [unwired: 10 in]
                n246 = call "日期字符串格式至时间格式转换(子VI).vi"("data[0]"=w389) -> ("time stamp"=w388:timestamp)  [unwired: 10 in]
                n247 = Build Array(w388) -> (w387:timestamp[])
                n248 = call "DateToHex.vi"("DATE"=w387) -> ("数组"=w386:u16[])  [unwired: 10 in]
              }
            }
            n249 = Build Array (concatenate)(w375, w374) -> (w373:u16[])
            n250 = call "Modbus Master.vi"("starting address"=w372, "holding register values"=w373, "读取写入选择"="写入", "Unit ID"=u8 1) -> ()  [unwired: 6 in, 6 out]
          }
          frame #1 {
            n251 = Wait (ms)(milliseconds to wait=u32 3000 ("等待时间（毫秒）")) -> ()  [unwired: 1 out]
          }
          frame #2 {
            n252 = global write "全局1.vi" "table元素"("反控命令" ("新元素/子数组")) -> ()
            n253 = call "Modbus Master.vi"("starting address"=w437, "holding register values"=u16[] [0], "读取写入选择"="写入", "Unit ID"=u8 1) -> ()  [unwired: 6 in, 6 out]
          }
        }
      }
    }
    frame "3040" {
      n254 = global write "全局1.vi" "table元素"("提取现场系统信息" ("新元素/子数组")) -> ()
    }
    frame "3041" {
      n255 = call "数据表比对.vi"("table输入"="环境参数" ("新元素/子数组")) -> ("columns输出"=w441:string[], "待发送数据"=w443:string[][])  [unwired: 7 in, 2 out]
      n256 = global write "全局 环境参数.vi" "环境参数"(w443) -> ()
      n257 = global write "全局 环境参数.vi" "columns输出"(w441) -> ()
      n258 = global write "全局1.vi" "table元素"("提取经纬度环境信息" ("新元素/子数组")) -> ()
    }
    frame "3042" {
      # "反控指令"
      # "反控指令\n切换运行模式"
      # "发命令给中控"
      # "0维护，1常规，2应急，3质控"
      n259 = global write "全局1.vi" "table元素"("反控命令" ("新元素/子数组")) -> ()
      n260 = Search/Split String(string=w459, search string/char (-)="RunMode" ("搜索字符串/字符(-)")) -> (match + rest of string=w456:string)  [unwired: 1 in, 2 out]
      n261 = String Subset(string=w456, offset (0)=8 ("偏移量(0)"), length (rest)=1 ("长度（剩余）")) -> (substring=w453:string)
      n262 = case shown="\"0\", 默认" w453 {
        tunnel: [u16 0 ("新元素/子数组") u16 1 ("新元素/子数组") u16 2 ("新元素/子数组") u16 3 ("新元素/子数组")] -> w449
        frame "0", Default {
        }
        frame "1" {
        }
        frame "2" {
        }
        frame "3" {
        }
      }
      n263 = Insert Into Array(array=u16[] [] ("holding register values"), index=0 ("索引"), new element=w449) -> (w450:u16[])
      n264 = call "Modbus Master.vi"("starting address"=u16 0, "holding register values"=w450, "读取写入选择"="写入", "Unit ID"=u8 1) -> ()  [unwired: 6 in, 6 out]
    }
    frame "3043" {
      n265 = flat-sequence {
        frame #0 {
          n266 = global write "全局1.vi" "table元素"("反控命令" ("新元素/子数组")) -> ()
        }
        frame #1 {
          n267 = call <vilib>:"System Exec.vi"("command line"="cmd /c shutdown/r") -> ("error out"=w465:errorcluster)  [unwired: 7 in, 3 out]
          n268 = call <vilib>:"Clear Errors.vi"("error in (no error)"=w465) -> ()  [unwired: 5 in, 2 out]
        }
      }
    }
    frame "3044" {
      n269 = flat-sequence {
        frame #0 {
          # "反控指令"
          # "发命令给中控"
          n270 = call "Modbus Master.vi"("starting address"=u16 2, "holding register values"=u16[] [1], "读取写入选择"="写入", "Unit ID"=u8 1) -> ()  [unwired: 6 in, 6 out]
        }
        frame #1 {
          # "反控指令\n单次测量"
          n271 = Wait (ms)(milliseconds to wait=u32 3000 ("等待时间（毫秒）")) -> ()  [unwired: 1 out]
        }
        frame #2 {
          n272 = global write "全局1.vi" "table元素"("反控命令" ("新元素/子数组")) -> ()
          n273 = call "Modbus Master.vi"("starting address"=u16 2, "holding register values"=u16[] [0], "读取写入选择"="写入", "Unit ID"=u8 1) -> ()  [unwired: 6 in, 6 out]
        }
      }
    }
    frame "3045", "3046" {
      n274 = flat-sequence {
        frame #0 {
          # "发命令给中控"
          n275 = call "Modbus Master.vi"("starting address"=u16 3, "holding register values"=u16[] [1], "读取写入选择"="写入", "Unit ID"=u8 1) -> ()  [unwired: 6 in, 6 out]
        }
        frame #1 {
          # "反控指令"
          # "反控指令\n急停"
          # "3045"
          n276 = Wait (ms)(milliseconds to wait=u32 3000 ("等待时间（毫秒）")) -> ()  [unwired: 1 out]
        }
        frame #2 {
          n277 = global write "全局1.vi" "table元素"("反控命令" ("新元素/子数组")) -> ()
          n278 = call "Modbus Master.vi"("starting address"=u16 3, "holding register values"=u16[] [0], "读取写入选择"="写入", "Unit ID"=u8 1) -> ()  [unwired: 6 in, 6 out]
        }
      }
    }
    frame "3056" {
      # "发回给平台"
      # "设置测量时间间隔"
      # "发命令给中控"
      n279 = global write "全局1.vi" "table元素"("反控命令" ("新元素/子数组")) -> ()
      n280 = Search/Split String(string=w498, search string/char (-)="RunInterval" ("搜索字符串/字符(-)")) -> (match + rest of string=w494:string)  [unwired: 1 in, 2 out]
      n281 = Decimal String To Number(string=w494, offset=12 ("偏移量(0)")) -> (number=w490:i32)  [unwired: 1 in, 1 out]
      n282 = Insert Into Array(array=u16[] [] ("holding register values"), index=0 ("索引"), new element=w490) -> (w489:u16[])
      n283 = call "Modbus Master.vi"("starting address"=u16 14, "holding register values"=w489, "读取写入选择"="写入", "Unit ID"=u8 1) -> ()  [unwired: 6 in, 6 out]
    }
    frame "3080", "3081", "3082", "3083", "3084", "3085", "3086" {
      n284 = flat-sequence {
        tunnel: w499 -> [w507]
        tunnel: [w505] -> w502
        tunnel: w500 -> [w504]
        tunnel: w502 -> [w532]
        tunnel: [w532] -> w501
        tunnel: w501 -> [w537]
        tunnel: [w534] -> _
        frame #0 {
          # "30 启动标液核查  1CODmn  2 氨氮  3总磷  4总氮  5CODCr\n31 加标回收\n32 平行样测试\n33 零点核查\n34 跨度核查\n35 校零\n36 校标"
          # "1CODmn  2 氨氮  3总磷  4总氮  5CODCr"
          # "启动单台仪器标液核查"
          # "发命令给中控"
          n285 = case shown="\"3081\"" w507 {
            tunnel: [u16 99 ("starting address") u16 30 ("starting address") u16 31 ("starting address") u16 32 ("starting address") u16 33 ("starting address") u16 34 ("starting address") u16 35 ("starting address") u16 36 ("starting address")] -> w505
            frame "", Default {
            }
            frame "3080" {
            }
            frame "3081" {
            }
            frame "3082" {
            }
            frame "3083" {
            }
            frame "3084" {
            }
            frame "3085" {
            }
            frame "3086" {
            }
          }
          n286 = Search/Split String(string=w504, search string/char (-)="PolId" ("搜索字符串/字符(-)")) -> (match + rest of string=w512:string)  [unwired: 1 in, 2 out]
          n287 = String Subset(string=w512, offset (0)=6 ("偏移量(0)"), length (rest)=6 ("长度（剩余）")) -> (substring=w509:string)
          n288 = case shown="\"w01019\"" w509 {
            tunnel: [0 ("长度（剩余）") 1 ("长度（剩余）") 2 ("长度（剩余）") 3 ("长度（剩余）") 4 ("长度（剩余）") 5 ("长度（剩余）")] -> w508
            frame "", Default {
            }
            frame "w01019" {
            }
            frame "w21003" {
            }
            frame "w21011" {
            }
            frame "w21001" {
            }
            frame "w01018" {
            }
          }
          n289 = Insert Into Array(array=u16[] [] ("holding register values"), index=0 ("索引"), new element=w508) -> (w513:u16[])
          n290 = call "Modbus Master.vi"("starting address"=w505, "holding register values"=w513, "读取写入选择"="写入", "Unit ID"=u8 1) -> ()  [unwired: 6 in, 6 out]
        }
        frame #1 {
          n291 = Wait (ms)(milliseconds to wait=u32 3000 ("等待时间（毫秒）")) -> ()  [unwired: 1 out]
        }
        frame #2 {
          n292 = global write "全局1.vi" "table元素"("反控命令" ("新元素/子数组")) -> ()
          n293 = call "Modbus Master.vi"("starting address"=w537, "holding register values"=u16[] [0], "读取写入选择"="写入", "Unit ID"=u8 1) -> ("error out"=w534:errorcluster)  [unwired: 6 in, 5 out]
        }
      }
    }
    frame "3200" {
      # "启动剖面水样测试"
      n294 = flat-sequence {
        frame #0 {
          # "反控指令"
          # "发命令给中控"
          n295 = call "Modbus Master.vi"("starting address"=u16 6, "holding register values"=u16[] [1], "读取写入选择"="写入", "Unit ID"=u8 1) -> ()  [unwired: 6 in, 6 out]
        }
        frame #1 {
          # "反控指令\n单次测量"
          n296 = Wait (ms)(milliseconds to wait=u32 3000 ("等待时间（毫秒）")) -> ()  [unwired: 1 out]
        }
        frame #2 {
          n297 = global write "全局1.vi" "table元素"("反控命令" ("新元素/子数组")) -> ()
          n298 = call "Modbus Master.vi"("starting address"=u16 6, "holding register values"=u16[] [0], "读取写入选择"="写入", "Unit ID"=u8 1) -> ()  [unwired: 6 in, 6 out]
        }
      }
    }
    frame "3201" {
      # "开启摄像头电源"
      n299 = flat-sequence {
        frame #0 {
          # "反控指令"
          # "发命令给中控"
          n300 = call "Modbus Master.vi"("starting address"=u16 7, "holding register values"=u16[] [1], "读取写入选择"="写入", "Unit ID"=u8 1) -> ()  [unwired: 6 in, 6 out]
        }
        frame #1 {
          # "反控指令\n单次测量"
          n301 = Wait (ms)(milliseconds to wait=u32 3000 ("等待时间（毫秒）")) -> ()  [unwired: 1 out]
        }
        frame #2 {
          n302 = global write "全局1.vi" "table元素"("反控命令" ("新元素/子数组")) -> ()
          n303 = call "Modbus Master.vi"("starting address"=u16 7, "holding register values"=u16[] [0], "读取写入选择"="写入", "Unit ID"=u8 1) -> ()  [unwired: 6 in, 6 out]
        }
      }
    }
  }
  "反控命令错误？" <- w2
  n304 = case shown="假" w2 {
    tunnel: w1 -> [w560 _]
    frame False {
      n305 = global write "全局 反控命令枚举.vi" "是否判断反馈？"(w560) -> ()
    }
    frame True {
    }
  }
